vi "Generate Voltage Signal.vi"   [LabVIEW 2024]
uses:
  <vilib>/measure/NI_MABase.lvlib
  <vilib>/measure/NI_MAPro.lvlib
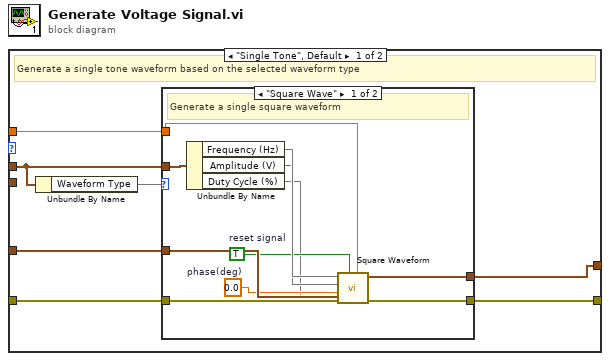
[diagram p0: block diagram]
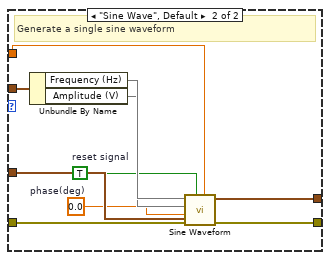
[diagram p2: hidden frame]
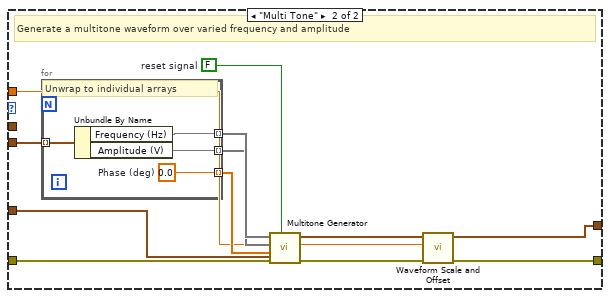
[diagram p3: hidden frame]
diagram:
  n1 = case shown="\"Single Tone\", Default" {
    selector: _ -> [_ _]
    tunnel: _ -> [w6 w40]
    tunnel: [w5 w32] -> _
    tunnel: [w4 w29] -> _
    tunnel: _ -> [w3 w39]
    tunnel: _ -> [w2 _]
    tunnel: _ -> [_ w38]
    tunnel: _ -> [w1 w30]
    frame "Single Tone", Default {
      # "Generate a single tone waveform based on the selected waveform type"
      n2 = Unbundle By Name(w2) -> ("Waveform Type"=w7)
      n3 = case shown="\"Square Wave\"" w7 {
        tunnel: w6 -> [w18 w28]
        tunnel: w2 -> [w16 w26]
        tunnel: w3 -> [w17 w27]
        tunnel: [w10 w21] -> w4
        tunnel: [w9 w20] -> w5
        tunnel: w1 -> [w8 w19]
        frame "Square Wave" {
          w12 = TRUE  # reset signal
          w13 = 0.0  # phase(deg)
          # "Generate a single square waveform"
          n4 = Unbundle By Name(w16) -> ("Frequency (Hz)"=w15, "Amplitude (V)"=w14, "Duty Cycle (%)"=w11)
          n5 = call <vilib>:"Square Waveform.vi"("duty cycle (%)"=w11, "offset"=w8, "sampling info"=w17, "reset signal"=w12, "error in (no error)"=w18, "phase"=w13, "amplitude"=w14, "frequency"=w15) -> ("error out"=w9:errorcluster, "signal out"=w10:waveform(dbl))  [unwired: 2 in]
        }
        frame "Sine Wave", Default {
          w22 = TRUE  # reset signal
          w23 = 0.0  # phase(deg)
          # "Generate a single sine waveform"
          n6 = Unbundle By Name(w26) -> ("Frequency (Hz)"=w25, "Amplitude (V)"=w24)
          n7 = call <vilib>:"Sine Waveform.vi"("offset"=w19, "sampling info"=w27, "reset signal"=w22, "error in (no error)"=w28, "phase"=w23, "amplitude"=w24, "frequency"=w25) -> ("error out"=w20:errorcluster, "signal out"=w21:waveform(dbl))  [unwired: 3 in]
        }
      }
    }
    frame "Multi Tone" {
      w34 = FALSE  # reset signal
      # "Generate a multitone waveform over varied frequency and amplitude"
      n8 = for {
        tunnel: w38 -> [w44] mode=indexing
        tunnel: [w43] -> w37 mode=indexing
        tunnel: [w42] -> w36 mode=indexing
        tunnel: [w41] -> w35 mode=indexing
        w41 = 0.0  # Phase (deg)
        # "Unwrap to individual arrays"
        n9 = Unbundle By Name(w44) -> ("Frequency (Hz)"=w43, "Amplitude (V)"=w42)
      }
      n10 = call <vilib>:"Multitone Generator.vi"("sampling info"=w39, "reset signal"=w34, "error in (no error)"=w40, "tone phases"=w35, "tone amplitudes"=w36, "tone frequencies"=w37) -> ("error out"=w33:errorcluster, "signal out"=w31:waveform(dbl))  [unwired: 2 in, 2 out]
      n11 = call <vilib>:"Waveform Scale and Offset.vi"("error in (no error)"=w33, "offset"=w30, "waveform in"=w31) -> ("error out"=w32:errorcluster, "waveform out"=w29:waveform(dbl))  [unwired: 7 in]
    }
  }
